vi "GetQMC_GetQMCA.vi"(0 "System no.":i32=1 min=1 step=1, 1 "Function":enum16{"GetQMC", "GetQMCA"}(ring), 2 "Axis":u8, 3 "Command":u8, 5 "error in":errorcluster, 6 "Parameter":u16) -> (14 "DLL I32 Return value":i32, 15 "Result":i32, 19 "error out":errorcluster)   [LabVIEW 2026]
doc: "This VI calls the GetQMC or GetQMCA function in the GCSTranslator.dll. GCSTranslator.dll and the corresponding system specific GCS DLL must be installed. The VI reads the system name from Global 2 (Array).vi and calls the corresponding DLL function. Parameter is only valid for GetQMCA. When using as a sub-VI, take special care to use the correct data representation when connecting values to the input terminals. If coercion dots appear at the terminals, the VI may not function correctly."
uses:
  Global1.vi
  GeneralCommands/Global2 (Array).vi
panel:
  # "This vi calls the GetQMC or GetQMCA function in the \nGCSTranslator.dll. GCSTranslator.dll and the corresponding \nsystem specific GCS DLL must be installed. The VI reads \nthe system name from Global 2 (Array) and calls the corres-\nponding DLL function. Parameter is only valid for GetQMCA."
  # "General inputs:"
  # "Function specific inputs:"
  # "Only valid for GetQMCA:"
  # "Error handling:"
  # "DLL output:"
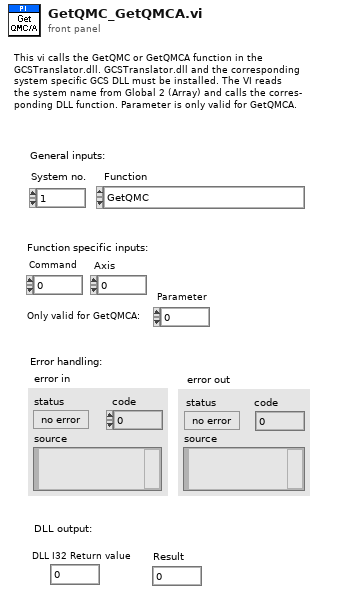
[diagram p1: front panel]
types:
  T1 = typedef "Controller names.ctl" = enum16{"None", "Analog", "C-702", "C-413", "C-414", "C-843", "C-843.PM", "C-844", "C-848", "C-865", "C-866", "C-867", "C-877", "C-880", "C-884", "C-885", "C-886", "C-887", "C-891", "E-135", "E-516", "E-517", "E-518", "E-709", "E-710", "E-712", "E-725", "E-727", "E-753", "E-754", "E-755", "E-761", "E-816", "E-861", "E-870", "E-871", "E-872", "E-873", "E-874", "F-206", "HydraPollux", "M-840", "M-850", "M-8X0", "Mercury", "Mercury_GCS", "PI_GCS2"}
  T2 = cluster{"Conn. axes":string[], "Controller name":T1}[]
  T3 = cluster{"Conn. axes":string[], "Controller name":T1}
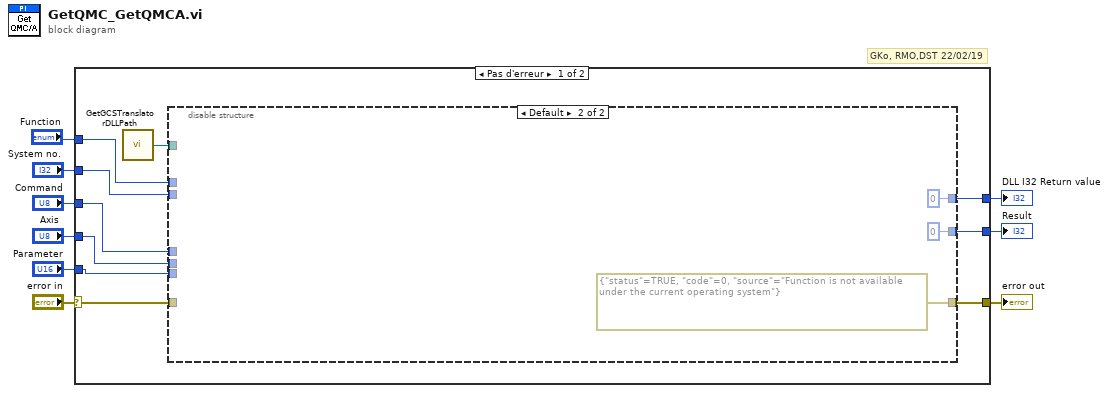
[diagram p0: block diagram]
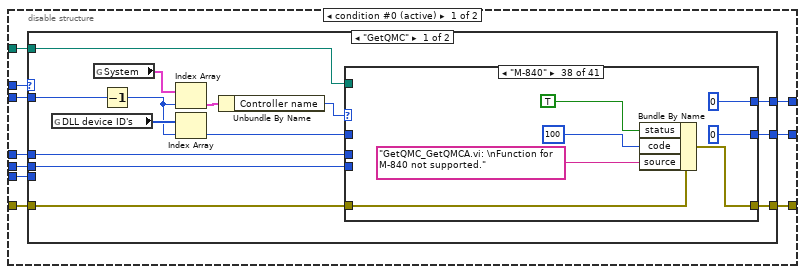
[diagram p2: hidden frame]
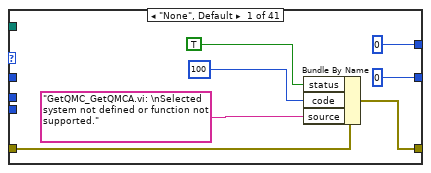
[diagram p3: hidden frame]
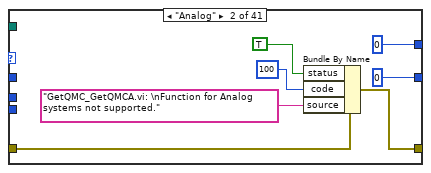
[diagram p4: hidden frame]
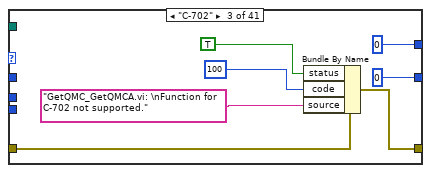
[diagram p5: hidden frame]
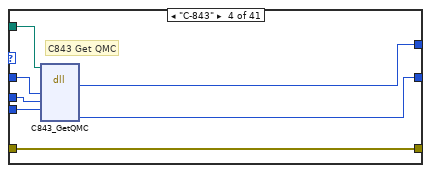
[diagram p6: hidden frame]
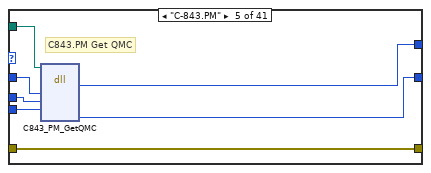
[diagram p7: hidden frame]
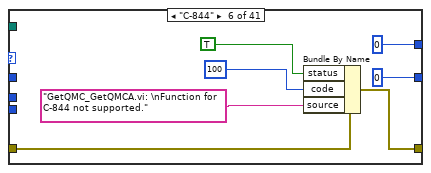
[diagram p8: hidden frame]
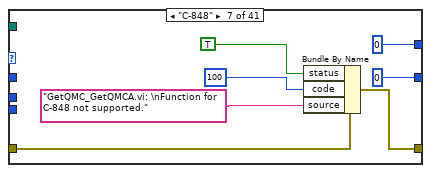
[diagram p9: hidden frame]
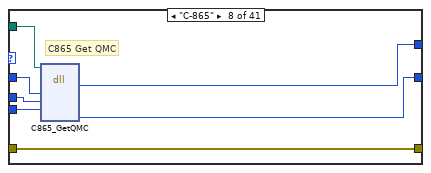
[diagram p10: hidden frame]
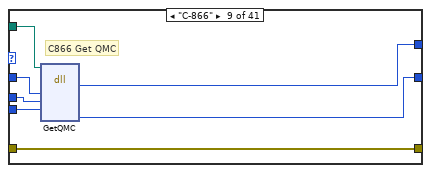
[diagram p11: hidden frame]
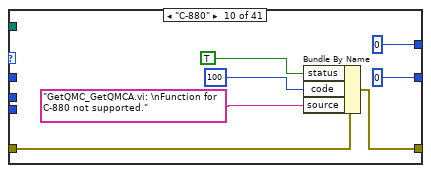
[diagram p12: hidden frame]
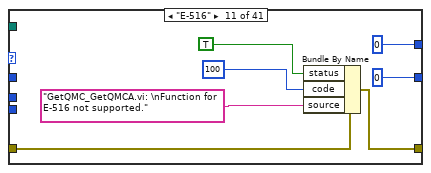
[diagram p13: hidden frame]
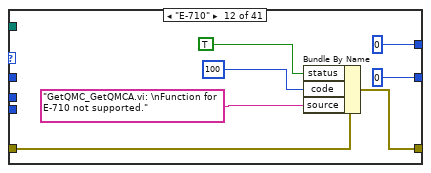
[diagram p14: hidden frame]
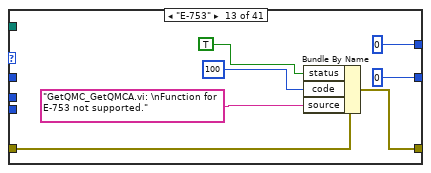
[diagram p15: hidden frame]
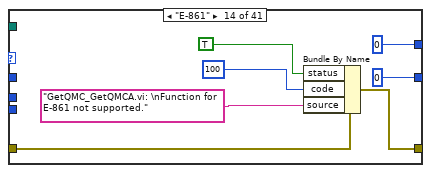
[diagram p16: hidden frame]
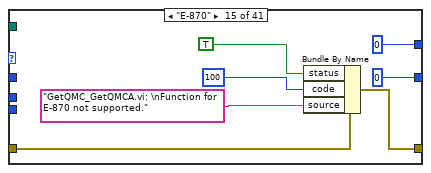
[diagram p17: hidden frame]
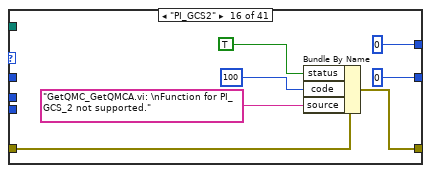
[diagram p18: hidden frame]
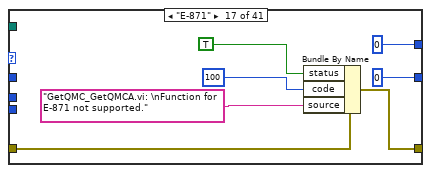
[diagram p19: hidden frame]
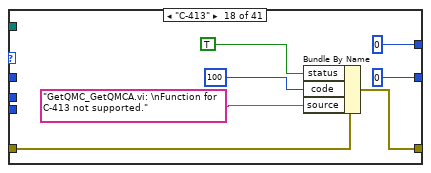
[diagram p20: hidden frame]
diagram:
  # "GKo, RMO,DST 22/02/19"
  n1 = case shown="Pas d'erreur" "error in" {
    selector: "error in" -> [w13 w507]
    tunnel: [w19 w507] -> w9
    tunnel: [w18 0] -> w8
    tunnel: "Command" -> [w17 _]
    tunnel: "Axis" -> [w16 _]
    tunnel: "Parameter" -> [w15 _]
    tunnel: [w14 0] -> w7
    tunnel: "System no." -> [w12 _]
    tunnel: "Function" -> [w11 _]
    frame No Error {
      n2 = call "GetGCSTranslatorDLLPath.vi"() -> ("DLL path"=w10:path)  [unwired: 1 in]
      n3 = disable-structure shown="Default" {
        disable-tunnel: w11 -> [w29 _]
        disable-tunnel: [w28 errorcluster {"status"=TRUE, "code"=0, "source"="Function is not available under the current operating system"} ("error IO")] -> w19
        disable-tunnel: [w27 0 ("return type")] -> w18
        disable-tunnel: w12 -> [w26 _]
        disable-tunnel: w17 -> [w25 _]
        disable-tunnel: w16 -> [w24 _]
        disable-tunnel: w15 -> [w23 _]
        disable-tunnel: [w22 0 ("lParam2")] -> w14
        disable-tunnel: w13 -> [w21 _]
        disable-tunnel: w10 -> [w20 _]
        frame condition #0 (active) {
          n4 = case shown="\"GetQMC\"" w29 {
            tunnel: w26 -> [w42 w344]
            tunnel: w21 -> [w36 w337]
            tunnel: [w35 w336] -> w28
            tunnel: [w43 w345] -> w27
            tunnel: w25 -> [w39 w341]
            tunnel: w24 -> [w38 w340]
            tunnel: w23 -> [_ w339]
            tunnel: [w37 w338] -> w22
            tunnel: w20 -> [w30 w331]
            frame "GetQMC" {
              n5 = global read "Global1.vi" "DLL device ID's"() -> (w41:i32[])
              n6 = global read "Global2 (Array).vi" "System"() -> (w34:T2)
              n7 = Decrement(x=w42) -> (x-1=w33:i32)
              n8 = Index Array(array=w34, index=w33) -> (element=w32:T3)
              n9 = Index Array(array=w41, index=w33) -> (element=w40:i32)
              n10 = Unbundle By Name(w32) -> ("Controller name"=w31:T1)
              n11 = case shown="\"M-840\"" w31 {
                tunnel: [0 0 0 w71 w78 0 0 w99 w106 0 0 0 0 0 0 0 0 0 0 0 0 0 0 0 0 0 0 0 0 0 0 0 0 0 0 0 0 0 0 0 0] -> w43
                tunnel: w40 -> [_ _ _ w70 w77 _ _ w98 w105 _ _ _ _ _ _ _ _ _ _ _ _ _ _ _ _ _ _ _ _ _ _ _ _ _ _ _ _ _ _ _ _]
                tunnel: w39 -> [_ _ _ w69 w76 _ _ w97 w104 _ _ _ _ _ _ _ _ _ _ _ _ _ _ _ _ _ _ _ _ _ _ _ _ _ _ _ _ _ _ _ _]
                tunnel: w38 -> [_ _ _ w68 w75 _ _ w96 w103 _ _ _ _ _ _ _ _ _ _ _ _ _ _ _ _ _ _ _ _ _ _ _ _ _ _ _ _ _ _ _ _]
                tunnel: [0 ("Result") 0 ("Result") 0 ("Result") w67 w74 0 ("Result") 0 ("Result") w95 w102 0 ("Result") 0 ("Result") 0 ("Result") 0 ("Result") 0 ("Result") 0 ("Result") 0 ("Result") 0 ("Result") 0 ("Result") 0 ("Result") 0 ("Result") 0 ("Result") 0 ("Result") 0 ("Result") 0 ("Result") 0 ("Result") 0 ("Result") 0 ("Result") 0 ("Result") 0 ("Result") 0 ("Result") 0 ("Result") 0 ("Result") 0 ("Result") 0 ("Result") 0 ("Result") 0 ("Result") 0 ("Result") 0 ("Result") 0 ("Result") 0 ("Result") 0 ("Result")] -> w37
                tunnel: [w44 w51 w58 w66 w73 w80 w87 w94 w101 w108 w115 w122 w128 w135 w142 w149 w156 w163 w170 w177 w184 w191 w198 w205 w212 w219 w226 w233 w240 w247 w254 w261 w268 w275 w282 w290 w297 w304 w311 w318 w324] -> w35
                tunnel: w36 -> [w45 w52 w59 w66 w73 w79 w86 w94 w101 w107 w114 w121 w129 w136 w143 w150 w157 w164 w171 w178 w185 w192 w199 w206 w213 w220 w227 w234 w241 w248 w255 w262 w269 w276 w283 w289 w296 w303 w310 w317 w325]
                tunnel: w30 -> [_ _ _ w65 w72 _ _ w93 w100 _ _ _ _ _ _ _ _ _ _ _ _ _ _ _ _ _ _ _ _ _ _ _ _ _ _ _ _ _ _ _ _]
                frame "None", Default {
                  n12 = Bundle By Name(cluster=w45, "status"=TRUE, "code"=100, "source"="GetQMC_GetQMCA.vi: \nSelected system not defined or function not supported.") -> (w44:errorcluster)
                }
                frame "Analog" {
                  n13 = Bundle By Name(cluster=w52, "status"=TRUE, "code"=100, "source"="GetQMC_GetQMCA.vi: \nFunction for Analog systems not supported.") -> (w51:errorcluster)
                }
                frame "C-702" {
                  n14 = Bundle By Name(cluster=w59, "status"=TRUE, "code"=100, "source"="GetQMC_GetQMCA.vi: \nFunction for C-702 not supported.") -> (w58:errorcluster)
                }
                frame "C-843" {
                  # "C843 Get QMC"
                  n15 = dll-call lib="T:/Entwicklung/HostSoftware/LabVIEW/GCSDrivers/source/GCS2LabVIEW/Low Level/GCSTranslator.dll" fn="C843_GetQMC"(path in=w65, "ID"=w70, "Cmd"=w69, "Axis"=w68) -> ("return type"=w71:i32, "Result"=w67:i32)  [unwired: 5 in, 3 out]
                }
                frame "C-843.PM" {
                  # "C843.PM Get QMC"
                  n16 = dll-call lib="T:/Entwicklung/HostSoftware/LabVIEW/GCSDrivers/source/GCS2LabVIEW/Low Level/GCSTranslator.dll" fn="C843_PM_GetQMC"(path in=w72, "ID"=w77, "Cmd"=w76, "Axis"=w75) -> ("return type"=w78:i32, "Result"=w74:i32)  [unwired: 5 in, 3 out]
                }
                frame "C-844" {
                  n17 = Bundle By Name(cluster=w79, "status"=TRUE, "code"=100, "source"="GetQMC_GetQMCA.vi: \nFunction for C-844 not supported.") -> (w80:errorcluster)
                }
                frame "C-848" {
                  n18 = Bundle By Name(cluster=w86, "status"=TRUE, "code"=100, "source"="GetQMC_GetQMCA.vi: \nFunction for C-848 not supported.") -> (w87:errorcluster)
                }
                frame "C-865" {
                  # "C865 Get QMC"
                  n19 = dll-call lib="T:/Entwicklung/HostSoftware/LabVIEW/GCSDrivers/source/GCS2LabVIEW/Low Level/GCSTranslator.dll" fn="C865_GetQMC"(path in=w93, "ID"=w98, "Cmd"=w97, "Axis"=w96) -> ("return type"=w99:i32, "Result"=w95:i32)  [unwired: 5 in, 3 out]
                }
                frame "C-866" {
                  # "C866 Get QMC"
                  n20 = dll-call lib="T:/Entwicklung/HostSoftware/LabVIEW/GCSDrivers/source/GCS2LabVIEW/Low Level/GCSTranslator.dll" fn="GetQMC"(path in=w100, "ID"=w105, "Cmd"=w104, "Axis"=w103) -> ("return type"=w106:i32, "Result"=w102:i32)  [unwired: 5 in, 3 out]
                }
                frame "C-880" {
                  n21 = Bundle By Name(cluster=w107, "status"=TRUE, "code"=100, "source"="GetQMC_GetQMCA.vi: \nFunction for C-880 not supported.") -> (w108:errorcluster)
                }
                frame "E-516" {
                  n22 = Bundle By Name(cluster=w114, "status"=TRUE, "code"=100, "source"="GetQMC_GetQMCA.vi: \nFunction for E-516 not supported.") -> (w115:errorcluster)
                }
                frame "E-710" {
                  n23 = Bundle By Name(cluster=w121, "status"=TRUE, "code"=100, "source"="GetQMC_GetQMCA.vi: \nFunction for E-710 not supported.") -> (w122:errorcluster)
                }
                frame "E-753" {
                  n24 = Bundle By Name(cluster=w129, "status"=TRUE, "code"=100, "source"="GetQMC_GetQMCA.vi: \nFunction for E-753 not supported.") -> (w128:errorcluster)
                }
                frame "E-861" {
                  n25 = Bundle By Name(cluster=w136, "status"=TRUE, "code"=100, "source"="GetQMC_GetQMCA.vi: \nFunction for E-861 not supported.") -> (w135:errorcluster)
                }
                frame "E-870" {
                  n26 = Bundle By Name(cluster=w143, "status"=TRUE, "code"=100, "source"="GetQMC_GetQMCA.vi: \nFunction for E-870 not supported.") -> (w142:errorcluster)
                }
                frame "PI_GCS2" {
                  n27 = Bundle By Name(cluster=w150, "status"=TRUE, "code"=100, "source"="GetQMC_GetQMCA.vi: \nFunction for PI_GCS_2 not supported.") -> (w149:errorcluster)
                }
                frame "E-871" {
                  n28 = Bundle By Name(cluster=w157, "status"=TRUE, "code"=100, "source"="GetQMC_GetQMCA.vi: \nFunction for E-871 not supported.") -> (w156:errorcluster)
                }
                frame "C-413" {
                  n29 = Bundle By Name(cluster=w164, "status"=TRUE, "code"=100, "source"="GetQMC_GetQMCA.vi: \nFunction for C-413 not supported.") -> (w163:errorcluster)
                }
                frame "Mercury_GCS" {
                  n30 = Bundle By Name(cluster=w171, "status"=TRUE, "code"=100, "source"="GetQMC_GetQMCA.vi: \nFunction for Mercury_GCS not supported.") -> (w170:errorcluster)
                }
                frame "C-867" {
                  n31 = Bundle By Name(cluster=w178, "status"=TRUE, "code"=100, "source"="GetQMC_GetQMCA.vi: \nFunction for C-867 not supported.") -> (w177:errorcluster)
                }
                frame "C-877" {
                  n32 = Bundle By Name(cluster=w185, "status"=TRUE, "code"=100, "source"="GetQMC_GetQMCA.vi: \nFunction for C-877 not supported.") -> (w184:errorcluster)
                }
                frame "C-891" {
                  n33 = Bundle By Name(cluster=w192, "status"=TRUE, "code"=100, "source"="GetQMC_GetQMCA.vi: \nFunction for C-891 not supported.") -> (w191:errorcluster)
                }
                frame "C-884" {
                  n34 = Bundle By Name(cluster=w199, "status"=TRUE, "code"=100, "source"="GetQMC_GetQMCA.vi: \nFunction for C-884 not supported.") -> (w198:errorcluster)
                }
                frame "C-885" {
                  n35 = Bundle By Name(cluster=w206, "status"=TRUE, "code"=100, "source"="GetQMC_GetQMCA.vi: \nFunction for C-885 not supported.") -> (w205:errorcluster)
                }
                frame "E-517" {
                  n36 = Bundle By Name(cluster=w213, "status"=TRUE, "code"=100, "source"="GetQMC_GetQMCA.vi: \nFunction for E-517 not supported.") -> (w212:errorcluster)
                }
                frame "E-518" {
                  n37 = Bundle By Name(cluster=w220, "status"=TRUE, "code"=100, "source"="GetQMC_GetQMCA.vi: \nFunction for E-518 not supported.") -> (w219:errorcluster)
                }
                frame "E-709" {
                  n38 = Bundle By Name(cluster=w227, "status"=TRUE, "code"=100, "source"="GetQMC_GetQMCA.vi: \nFunction for E-709 not supported.") -> (w226:errorcluster)
                }
                frame "E-712" {
                  n39 = Bundle By Name(cluster=w234, "status"=TRUE, "code"=100, "source"="GetQMC_GetQMCA.vi: \nFunction for E-712 not supported.") -> (w233:errorcluster)
                }
                frame "E-725" {
                  n40 = Bundle By Name(cluster=w241, "status"=TRUE, "code"=100, "source"="GetQMC_GetQMCA.vi: \nFunction for E-725 not supported.") -> (w240:errorcluster)
                }
                frame "E-727" {
                  n41 = Bundle By Name(cluster=w248, "status"=TRUE, "code"=100, "source"="GetQMC_GetQMCA.vi: \nFunction for E-727 not supported.") -> (w247:errorcluster)
                }
                frame "E-754" {
                  n42 = Bundle By Name(cluster=w255, "status"=TRUE, "code"=100, "source"="GetQMC_GetQMCA.vi: \nFunction for E-754 not supported.") -> (w254:errorcluster)
                }
                frame "E-873" {
                  n43 = Bundle By Name(cluster=w262, "status"=TRUE, "code"=100, "source"="GetQMC_GetQMCA.vi: \nFunction for E-873 not supported.") -> (w261:errorcluster)
                }
                frame "HydraPollux" {
                  n44 = Bundle By Name(cluster=w269, "status"=TRUE, "code"=100, "source"="GetQMC_GetQMCA.vi: \nFunction for Hydra/Pollux not supported.") -> (w268:errorcluster)
                }
                frame "E-755" {
                  n45 = Bundle By Name(cluster=w276, "status"=TRUE, "code"=100, "source"="GetQMC_GetQMCA.vi: \nFunction for E-755 not supported.") -> (w275:errorcluster)
                }
                frame "E-761" {
                  n46 = Bundle By Name(cluster=w283, "status"=TRUE, "code"=100, "source"="GetQMC_GetQMCA.vi: \nFunction for E-761 not supported.") -> (w282:errorcluster)
                }
                frame "E-816" {
                  n47 = Bundle By Name(cluster=w289, "status"=TRUE, "code"=100, "source"="GetQMC_GetQMCA.vi: \nFunction for E-816 not supported.") -> (w290:errorcluster)
                }
                frame "F-206" {
                  n48 = Bundle By Name(cluster=w296, "status"=TRUE, "code"=100, "source"="GetQMC_GetQMCA.vi: \nFunction for F-206 not supported.") -> (w297:errorcluster)
                }
                frame "M-840" {
                  n49 = Bundle By Name(cluster=w303, "status"=TRUE, "code"=100, "source"="GetQMC_GetQMCA.vi: \nFunction for M-840 not supported.") -> (w304:errorcluster)
                }
                frame "M-850" {
                  n50 = Bundle By Name(cluster=w310, "status"=TRUE, "code"=100, "source"="GetQMC_GetQMCA.vi: \nFunction for M-850 not supported.") -> (w311:errorcluster)
                }
                frame "M-8X0" {
                  n51 = Bundle By Name(cluster=w317, "status"=TRUE, "code"=100, "source"="GetQMC_GetQMCA.vi: \nFunction for M-8X0 not supported.") -> (w318:errorcluster)
                }
                frame "Mercury" {
                  n52 = Bundle By Name(cluster=w325, "status"=TRUE, "code"=100, "source"="GetQMC_GetQMCA.vi: \nFunction for Mercury not supported.") -> (w324:errorcluster)
                }
              }
            }
            frame "GetQMCA" {
              n53 = global read "Global1.vi" "DLL device ID's"() -> (w343:i32[])
              n54 = global read "Global2 (Array).vi" "System"() -> (w333:T2)
              n55 = Decrement(x=w344) -> (x-1=w335:i32)
              n56 = Index Array(array=w333, index=w335) -> (element=w334:T3)
              n57 = Index Array(array=w343, index=w335) -> (element=w342:i32)
              n58 = Unbundle By Name(w334) -> ("Controller name"=w332:T1)
              n59 = case shown="\"C-843\"" w332 {
                tunnel: [0 0 0 w374 w382 0 0 0 w411 w419 0 0 0 0 0 0 0 0 0 0 0 0] -> w345
                tunnel: w342 -> [_ _ _ w373 w381 _ _ _ w410 w418 _ _ _ _ _ _ _ _ _ _ _ _]
                tunnel: w341 -> [_ _ _ w372 w380 _ _ _ w409 w417 _ _ _ _ _ _ _ _ _ _ _ _]
                tunnel: w340 -> [_ _ _ w371 w379 _ _ _ w408 w416 _ _ _ _ _ _ _ _ _ _ _ _]
                tunnel: w339 -> [_ _ _ w370 w378 _ _ _ w407 w415 _ _ _ _ _ _ _ _ _ _ _ _]
                tunnel: [0 ("lParam2") 0 ("lParam2") 0 ("lParam2") w369 w377 0 ("lParam2") 0 ("lParam2") 0 ("lParam2") w406 w414 0 ("lParam2") 0 ("lParam2") 0 ("lParam2") 0 ("lParam2") 0 ("lParam2") 0 ("lParam2") 0 ("lParam2") 0 ("lParam2") 0 ("lParam2") 0 ("lParam2") 0 ("lParam2") 0 ("lParam2")] -> w338
                tunnel: w337 -> [w347 w354 w361 w368 w376 w383 w390 w397 w405 w413 w420 w427 w434 w441 w449 w456 w462 w469 w476 w483 w490 w498]
                tunnel: [w346 w353 w360 w368 w376 w384 w391 w398 w405 w413 w421 w428 w435 w442 w448 w455 w463 w470 w477 w484 w491 w497] -> w336
                tunnel: w331 -> [_ _ _ w367 w375 _ _ _ w404 w412 _ _ _ _ _ _ _ _ _ _ _ _]
                frame "None", Default {
                  n60 = Bundle By Name(cluster=w347, "status"=TRUE, "code"=100, "source"="GetQMC_GetQMCA.vi: \nSelected system not defined or function not supported.") -> (w346:errorcluster)
                }
                frame "Analog" {
                  n61 = Bundle By Name(cluster=w354, "status"=TRUE, "code"=100, "source"="GetQMC_GetQMCA.vi: \nFunction for Analog Systems not supported.") -> (w353:errorcluster)
                }
                frame "C-702" {
                  n62 = Bundle By Name(cluster=w361, "status"=TRUE, "code"=100, "source"="GetQMC_GetQMCA.vi: \nFunction for C-702 not supported.") -> (w360:errorcluster)
                }
                frame "C-843" {
                  # "C843 Get QMCA"
                  n63 = dll-call lib="T:/Entwicklung/HostSoftware/LabVIEW/GCSDrivers/source/GCS2LabVIEW/Low Level/GCSTranslator.dll" fn="C843_GetQMCA"(path in=w367, "ID"=w373, "Cmd"=w372, "Axis"=w371, "Param"=w370) -> ("return type"=w374:i32, "Result"=w369:i32)  [unwired: 6 in, 3 out]
                }
                frame "C-843.PM" {
                  # "C843.PM Get QMCA"
                  n64 = dll-call lib="T:/Entwicklung/HostSoftware/LabVIEW/GCSDrivers/source/GCS2LabVIEW/Low Level/GCSTranslator.dll" fn="C843_PM_GetQMCA"(path in=w375, "ID"=w381, "Cmd"=w380, "Axis"=w379, "Param"=w378) -> ("return type"=w382:i32, "Result"=w377:i32)  [unwired: 6 in, 3 out]
                }
                frame "C-844" {
                  n65 = Bundle By Name(cluster=w383, "status"=TRUE, "code"=100, "source"="GetQMC_GetQMCA.vi: \nFunction for C-844 not supported.") -> (w384:errorcluster)
                }
                frame "C-848" {
                  n66 = Bundle By Name(cluster=w390, "status"=TRUE, "code"=100, "source"="GetQMC_GetQMCA.vi: \nFunction for C-848 not supported.") -> (w391:errorcluster)
                }
                frame "PI_GCS2" {
                  n67 = Bundle By Name(cluster=w397, "status"=TRUE, "code"=100, "source"="GetQMC_GetQMCA.vi: \nFunction for PI_GCS_2 not supported.") -> (w398:errorcluster)
                }
                frame "C-865" {
                  # "C865 Get QMCA"
                  n68 = dll-call lib="T:/Entwicklung/HostSoftware/LabVIEW/GCSDrivers/source/GCS2LabVIEW/Low Level/GCSTranslator.dll" fn="C865_GetQMCA"(path in=w404, "ID"=w410, "Cmd"=w409, "Axis"=w408, "Param"=w407) -> ("return type"=w411:i32, "Result"=w406:i32)  [unwired: 6 in, 3 out]
                }
                frame "C-866" {
                  # "C866 Get QMCA"
                  n69 = dll-call lib="T:/Entwicklung/HostSoftware/LabVIEW/GCSDrivers/source/GCS2LabVIEW/Low Level/GCSTranslator.dll" fn="GetQMCA"(path in=w412, "ID"=w418, "Cmd"=w417, "Axis"=w416, "Param"=w415) -> ("return type"=w419:i32, "Result"=w414:i32)  [unwired: 6 in, 3 out]
                }
                frame "C-880" {
                  n70 = Bundle By Name(cluster=w420, "status"=TRUE, "code"=100, "source"="GetQMC_GetQMCA.vi: \nFunction for C-880 not supported.") -> (w421:errorcluster)
                }
                frame "E-516" {
                  n71 = Bundle By Name(cluster=w427, "status"=TRUE, "code"=100, "source"="GetQMC_GetQMCA.vi: \nFunction for E-516 not supported.") -> (w428:errorcluster)
                }
                frame "E-710" {
                  n72 = Bundle By Name(cluster=w434, "status"=TRUE, "code"=100, "source"="GetQMC_GetQMCA.vi: \nFunction for E-710 not supported.") -> (w435:errorcluster)
                }
                frame "E-753" {
                  n73 = Bundle By Name(cluster=w441, "status"=TRUE, "code"=100, "source"="GetQMC_GetQMCA.vi: \nFunction for E-753 not supported.") -> (w442:errorcluster)
                }
                frame "E-755" {
                  n74 = Bundle By Name(cluster=w449, "status"=TRUE, "code"=100, "source"="GetQMC_GetQMCA.vi: \nFunction for E-755 not supported.") -> (w448:errorcluster)
                }
                frame "E-761" {
                  n75 = Bundle By Name(cluster=w456, "status"=TRUE, "code"=100, "source"="GetQMC_GetQMCA.vi: \nFunction for E-761 not supported.") -> (w455:errorcluster)
                }
                frame "E-816" {
                  n76 = Bundle By Name(cluster=w462, "status"=TRUE, "code"=100, "source"="GetQMC_GetQMCA.vi: \nFunction for E-816 not supported.") -> (w463:errorcluster)
                }
                frame "F-206" {
                  n77 = Bundle By Name(cluster=w469, "status"=TRUE, "code"=100, "source"="GetQMC_GetQMCA.vi: \nFunction for F-206 not supported.") -> (w470:errorcluster)
                }
                frame "M-840" {
                  n78 = Bundle By Name(cluster=w476, "status"=TRUE, "code"=100, "source"="GetQMC_GetQMCA.vi: \nFunction for M-840 not supported.") -> (w477:errorcluster)
                }
                frame "M-850" {
                  n79 = Bundle By Name(cluster=w483, "status"=TRUE, "code"=100, "source"="GetQMC_GetQMCA.vi: \nFunction for M-850 not supported.") -> (w484:errorcluster)
                }
                frame "M-8X0" {
                  n80 = Bundle By Name(cluster=w490, "status"=TRUE, "code"=100, "source"="GetQMC_GetQMCA.vi: \nFunction for M-8X0 not supported.") -> (w491:errorcluster)
                }
                frame "Mercury" {
                  n81 = Bundle By Name(cluster=w498, "status"=TRUE, "code"=100, "source"="GetQMC_GetQMCA.vi: \nFunction for Mercury not supported.") -> (w497:errorcluster)
                }
              }
            }
          }
        }
        frame condition #1 {
        }
      }
    }
    frame Error {
    }
  }
  "error out" <- w9
  "DLL I32 Return value" <- w8
  "Result" <- w7
